vi "TRITON_Set Temperature.vi"(2 "error in (no error)":errorcluster, 3 "setpoint":dbl=0.1) -> (0 "error out":errorcluster)   [LabVIEW 2021]
panel:
  out "Response String":string
  in  "Mode":T1(ring)=enum."Immediate"
  in  "Bytes to Read":i32=5000
  in  "IP Address":string="192.168.0.2"
  in  "Remote Port":i32=33576
  in  "Timeout":i32=10000
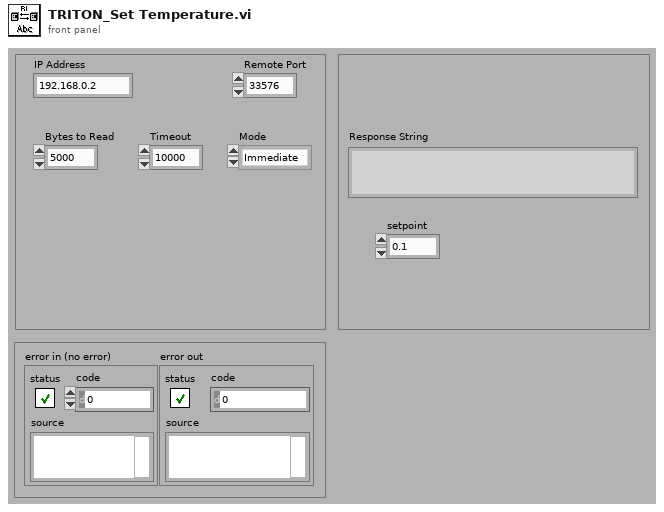
[diagram p1: front panel]
types:
  T1 = enum16{"Standard", "Buffered", "CRLF", "Immediate"}
  T2 = cluster{"Mode":enum16{"Standard", "Buffered", "CRLF", "Immediate"}, "Bytes to Read":i32, "IP Address":string, "Remote Port":i32, "Timeout":i32}
  T3 = cluster{"Mode":enum16{"Standard", "Buffered", "CRLF", "Immediate"}, "Bytes to Read":i32, "IP Address":string, "Remote Port":i32, "Timeout":i32, "connection ID":refnum<k5>}
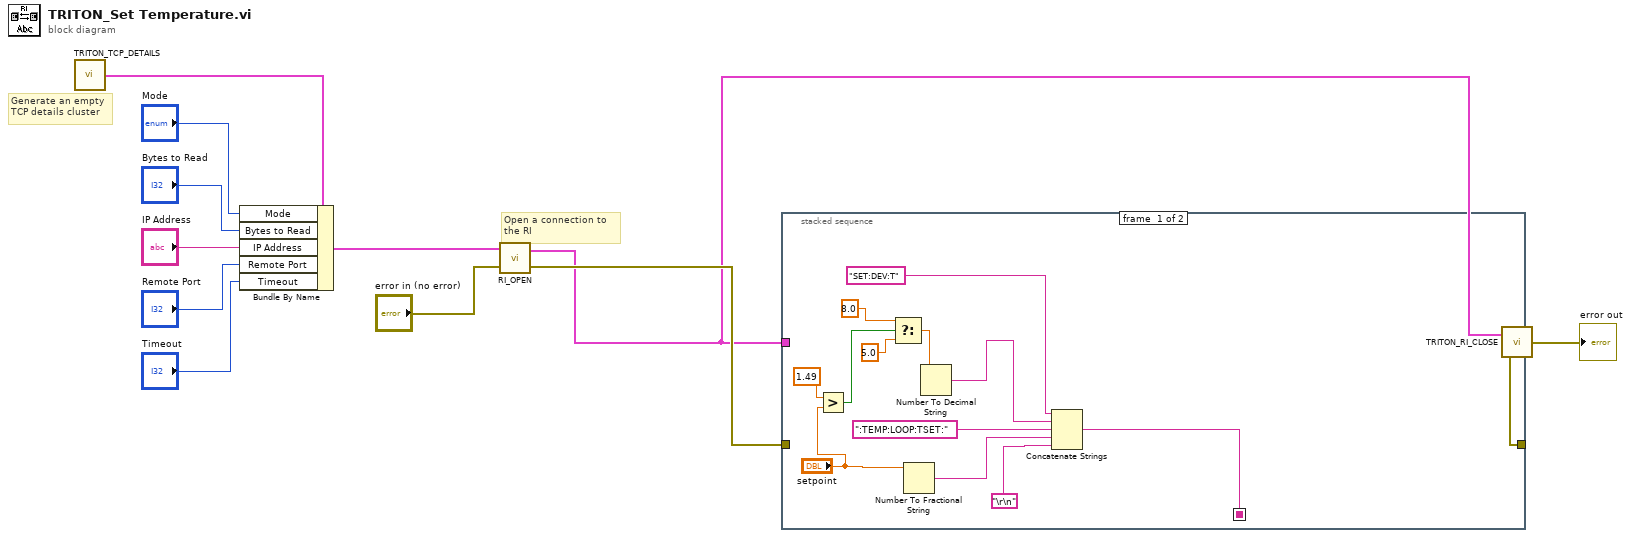
[diagram p0: block diagram]
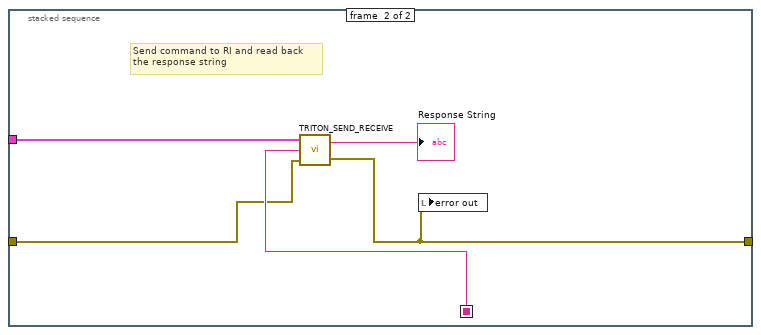
[diagram p2: hidden frame]
diagram:
  # "Open a connection to\nthe RI"
  # "Generate an empty\nTCP details cluster"
  n1 = call "TRITON_TCP_DETAILS.vi"() -> ("Cluster"=w12:T2)
  n2 = Bundle By Name(cluster=w12, "Mode"="Mode", "Bytes to Read"="Bytes to Read", "IP Address"="IP Address", "Remote Port"="Remote Port", "Timeout"="Timeout") -> (w10:T2)
  n3 = call "RI_OPEN.vi"("error in (no error)"="error in (no error)", "Cluster"=w10) -> ("error out"=w9:errorcluster, "output cluster"=w6:T3)
  n4 = stacked-sequence {
    seq-local: [w24 _] -> [_ w29]
    tunnel: w9 -> [_ w28]
    tunnel: [_ w27] -> w8
    tunnel: w6 -> [_ w26]
    frame #0 {
      n5 = Greater?(x=1.49, y="setpoint") -> (0:w21:bool)
      n6 = Select(t=8.0, s=w21, f=5.0) -> (s? t:f=w14:dbl)
      n7 = Number To Fractional String(number="setpoint") -> (F-format string=w16:string)  [unwired: 3 in]
      n8 = Number To Decimal String(number=w14) -> (decimal integer string=w13:string)  [unwired: 1 in]
      n9 = Concatenate Strings("SET:DEV:T", w13, ":TEMP:LOOP:TSET:", w16, "\r\n") -> (w24:string)
    }
    frame #1 {
      # "Send command to RI and read back\nthe response string"
      n10 = call "TRITON_SEND_RECEIVE.vi"("error in (no error)"=w28, "Command String"=w29, "Communication Cluster"=w26) -> ("error out"=w27:errorcluster, "Response String"=→"Response String":string)
      n11 = local write "error out"(w27) -> ()
    }
  }
  n12 = call "TRITON_RI_CLOSE.vi"("error in (no error)"=w8, "Communication Cluster"=w6) -> ("error out"=→"error out":errorcluster)
